vi "Send_SET_1BIT.vi"(8 "error in (no error)":errorcluster, 9 "Encender?":bool, 10 "Channel":u8, 11 "Serial Device in":refnum<class "Serial Device.lvclass">) -> (0 "error out":errorcluster, 2 "Response":string, 3 "Serial Device out":refnum<class "Serial Device.lvclass">)   [LabVIEW 2019, in "Serial Device.lvclass"]
uses:
  Serial Device.lvclass
  Serial Device.lvclass/Serial Device.ctl
  0713ec9a-b44c-44ab-a500-c5f2b92f772c.vi
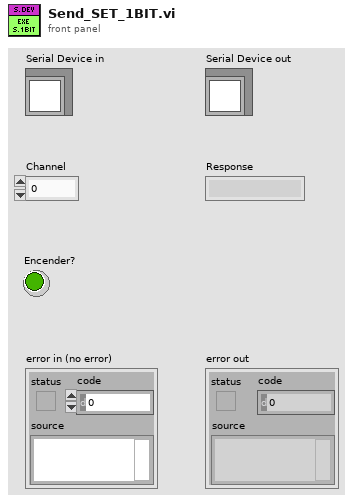
[diagram p1: front panel]
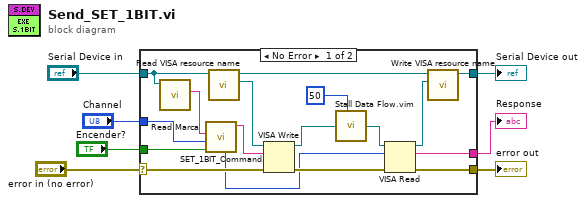
[diagram p0: block diagram]
diagram:
  n1 = case shown="No Error" "error in (no error)" {
    selector: "error in (no error)" -> [w22 w26]
    tunnel: [w18 w26] -> w6
    tunnel: [w14 w25] -> w4
    tunnel: "Serial Device in" -> [w24 w25]
    tunnel: "Channel" -> [w11 _]
    tunnel: [w13 _] -> w2
    tunnel: "Encender?" -> [w8 _]
    frame No Error {
      n2 = call "Read Marca.vi"("Serial Device in"=w24) -> ("Marca"=w12:string)  [unwired: 8 in, 2 out]
      n3 = call "SET_1BIT_Command.vi"("Encender?"=w8, "Canal"=w11, "Marca"=w12) -> ("Command"=w9:string, "Bytes Expected"=w10:u32)  [unwired: 5 in, 2 out]
      n4 = call "Read VISA resource name.vi"("Serial Device in"=w24) -> ("VISA resource name"=w23:refnum<visa-resource-name>, "Serial Device out"=w15:refnum<class "Serial Device.lvclass">)  [unwired: 8 in, 1 out]
      n5 = VISA Write(VISA resource name=w23, write buffer=w9, error in (no error)=w22) -> (VISA resource name out=w21:refnum<visa-resource-name>, error out=w19:errorcluster)  [unwired: 1 out]
      n6 = call "Stall Data Flow.vim"("value in"=w21, "milliseconds to wait"=u32 50) -> ("value out"=w20:refnum<visa-resource-name>)  [unwired: 1 out]
      n7 = VISA Read(VISA resource name=w20, byte count=w10, error in (no error)=w19) -> (VISA resource name out=w16:refnum<visa-resource-name>, read buffer=w13:string, error out=w18:errorcluster)  [unwired: 1 out]
      n8 = call "Write VISA resource name.vi"("VISA resource name"=w16, "Serial Device in"=w15) -> ("Serial Device out"=w14:refnum<class "Serial Device.lvclass">)  [unwired: 8 in, 1 out]
    }
    frame Error {
    }
  }
  "error out" <- w6
  "Serial Device out" <- w4
  "Response" <- w2
